vi "ShutDownWebpage.vi"(11 "address":string="192.168.68.70:53251") -> (0 "error out":errorcluster)   [LabVIEW 2026, in "WebPage Addon Shared.lvlib"]
uses:
  WebPage Addon Shared.lvlib
  gRPCWebPageInterface.lvlibp
panel:
  out "Response Data":T1
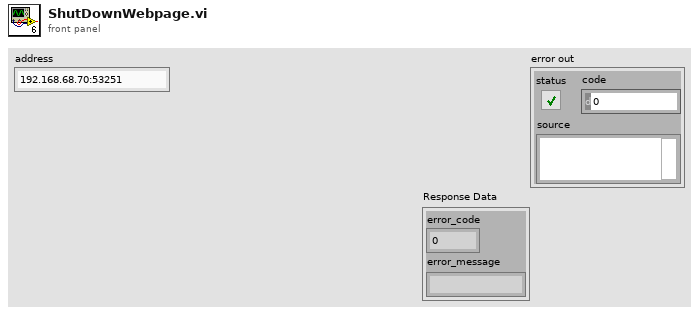
[diagram p1: front panel]
types:
  T1 = cluster{"error_code":i32, "error_message":string}
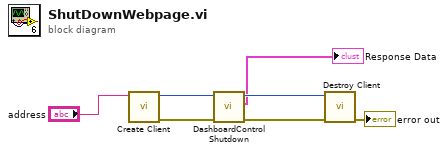
[diagram p0: block diagram]
diagram:
  n1 = call "Create Client.vi"("address"="address") -> ("error out"=w4:errorcluster, "gRPC ID Out"=w7:u64)  [unwired: 9 in]
  n2 = call "DashboardControl Shutdown.vi"("error in"=w4, "gRPC ID"=w7) -> ("error out"=w5:errorcluster, "Response Data"=→"Response Data":T1, "gRPC ID out"=w6:u64)  [unwired: 7 in]
  n3 = call "Destroy Client.vi"("error in"=w5, "gRPC ID"=w6) -> ("error out"=→"error out":errorcluster)  [unwired: 9 in]
